vi "Main.vi"() -> ()   [LabVIEW 2019, in "TemplateModule.lvlib"]
doc: "This VI is a template for all GUI VIs in TMOS. Be careful with colours, they may require updating."
uses:
  TemplateModule.lvlib
  Gui/Gui.TopBar.ctl
  Tools/controls/buttons/OK.ctl
  Tools/controls/buttons/Cancel.ctl
  Tools/controls/buttons/Reload.ctl
  Tools/controls/buttons/Save.ctl
  Action.ctl
  Gui/Gui.TopBar.Visibility.ctl
  Tools/CitTemplate/citTemplate.errData.ctl
  Tools/Tools.lvlib
panel:
  in  "Module top bar":T1
  # "version: 1.0"
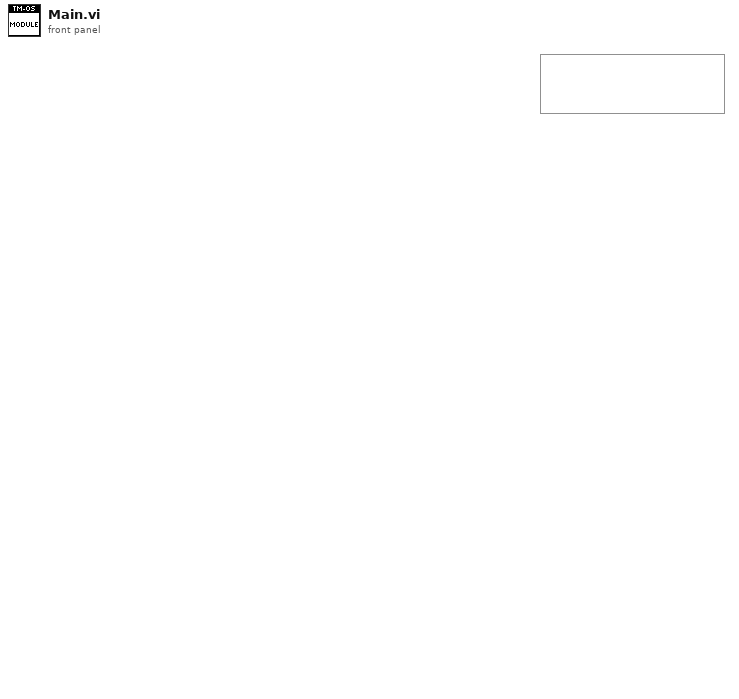
[diagram p1: front panel]
types:
  T1 = typedef "TemplateModule.lvlib/Gui.TopBar.ctl" = cluster{"OK":T2, "Cancel":T3, "Reload":T4, "Save":T5, "Module name":string}
  T2 = typedef "Tools.lvlib/OK.ctl" = bool
  T3 = typedef "Tools.lvlib/Cancel.ctl" = bool
  T4 = typedef "Tools.lvlib/Reload.ctl" = bool
  T5 = typedef "Tools.lvlib/Save.ctl" = bool
  T6 = typedef "TemplateModule.lvlib/Action.ctl" = enum32{"idle", "constructor", "destructor", "--- Module.Gui ---", "Translate.Gui", "update"}
  T7 = typedef "Tools.lvlib/citTemplate.errData.ctl" = cluster{"action":string, "error":errorcluster}
  T8 = typedef "Tools.lvlib/citTemplate.notifierHandle.ctl" = refnum<notifier>
  T9 = typedef "TemplateModule.lvlib/Gui.TopBar.Visibility.ctl" = cluster{"OK":bool, "Cancel":bool, "Reload":bool, "Save":bool, "Module name":bool}
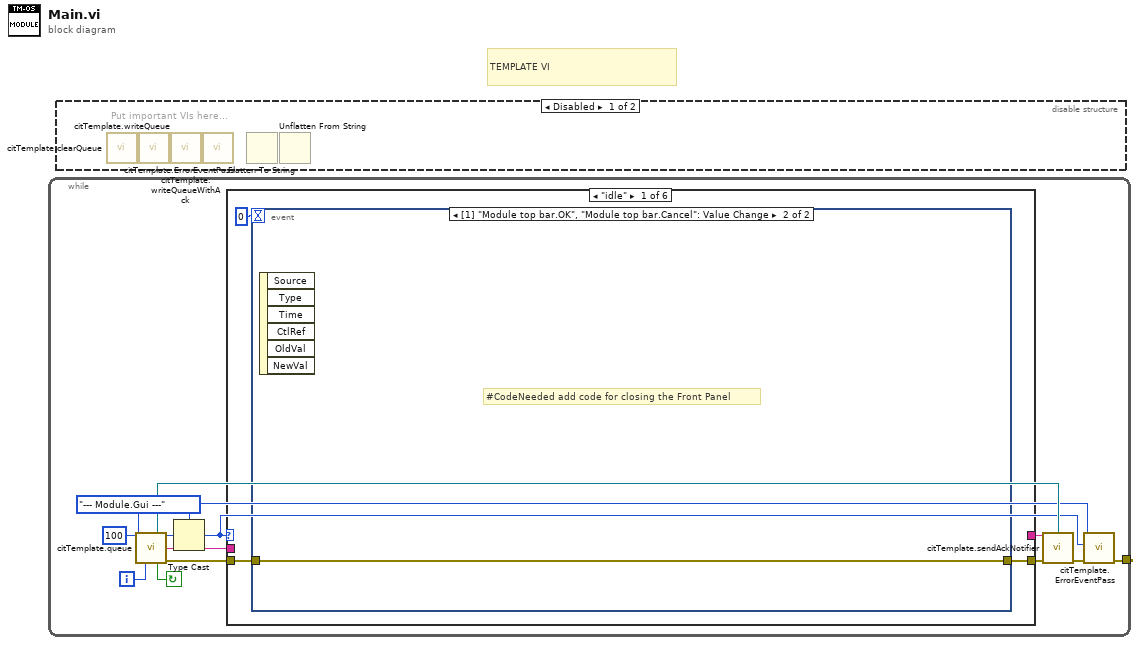
[diagram p0: block diagram]
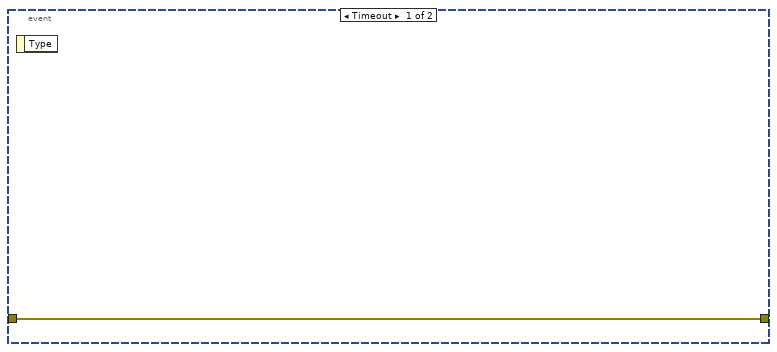
[diagram p3: hidden frame]
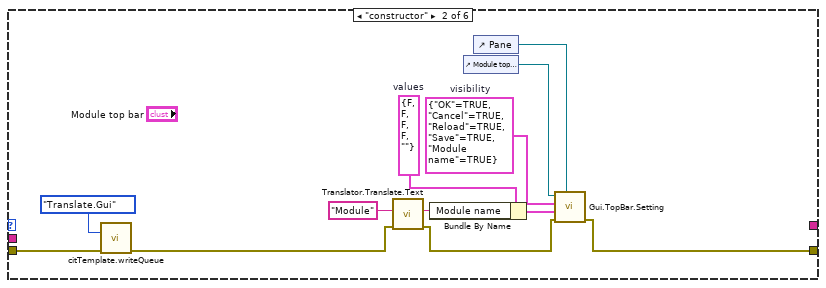
[diagram p4: hidden frame]
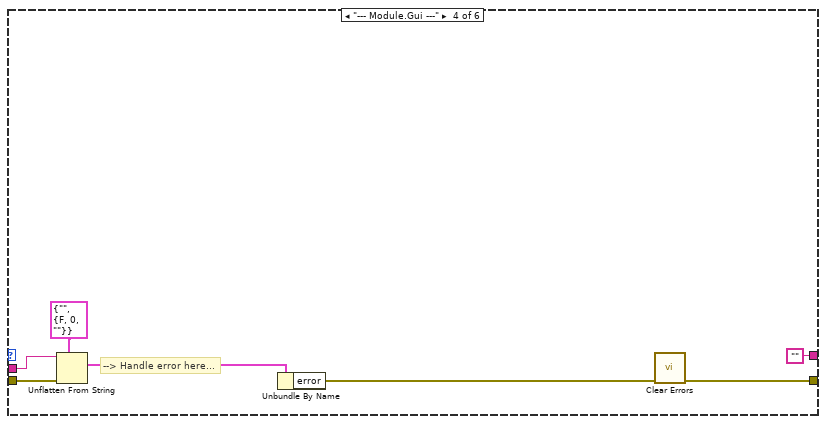
[diagram p6: hidden frame]
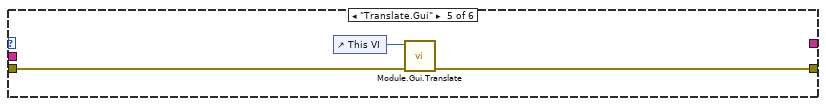
[diagram p7: hidden frame]
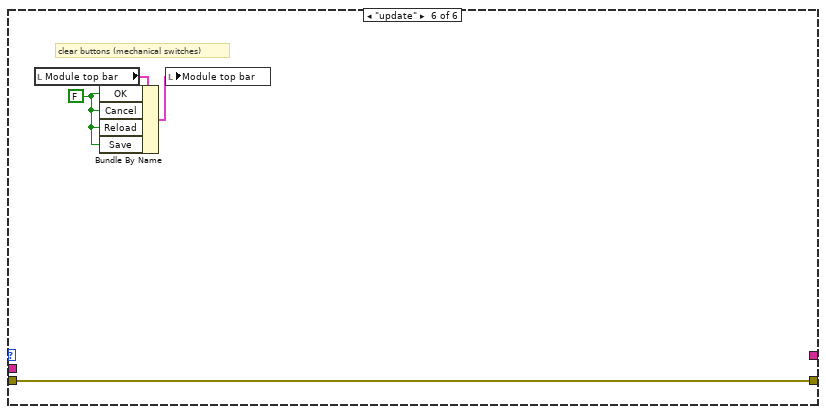
[diagram p8: hidden frame]
diagram:
  # "TEMPLATE VI"
  n1 = while {
    tunnel: [w2] -> _
    i -> [w8]
    stop <- w9 continue-if-true
    w1 = Action."--- Module.Gui ---" ("Action")
    n2 = call "citTemplate.queue.vi"("ms timeout (250 ms)"=100, "event enum"=w1, "iteration (-1)"=w8) -> ("notifierHandle out"=w6:T8, "event out"=w12:u32, "(flatten) data out"=w11:string, "continue"=w9:bool, "error out"=w10:errorcluster)  [unwired: 2 in, 6 out]
    n3 = Type Cast(type=w1, x=w12) -> (*(type *) &x=w3:T6)
    n4 = case shown="\"idle\"" w3 {
      tunnel: w11 -> [_ _ _ w37 _ _]
      tunnel: w10 -> [w14 w29 w30 w36 w39 w44]
      tunnel: [w13 w22 w30 w34 w38 w44] -> w4
      tunnel: [_ _ _ "" _ _] -> w5
      frame "idle" {
        n5 = event shown="[1] \"Module top bar.OK\", \"Module top bar.Cancel\": Value Change" {
          selector: _ -> [_ _]
          dyn-events: _ -> [_ _]
          timeout: 0 -> [_ _]
          tunnel: [w16 w17] -> w13
          tunnel: w14 -> [w16 w17]
          event Timeout {
            n6 = event-data() -> ()  [unwired: 1 in, 1 out]
          }
          event Value Change {
            # "#CodeNeeded add code for closing the Front Panel"
            n7 = event-data() -> ()  [unwired: 1 in, 6 out]
          }
        }
      }
      frame "constructor" {
        w26 = T1 {"OK"=FALSE, "Cancel"=FALSE, "Reload"=FALSE, "Save"=FALSE, "Module name"=""}  # values
        w27 = T9 {"OK"=TRUE, "Cancel"=TRUE, "Reload"=TRUE, "Save"=TRUE, "Module name"=TRUE}  # visibility
        n8 = call "citTemplate.writeQueue.vi"("event in (if not connected:all statemachine with data event)"=Action."Translate.Gui" ("Action"), "error in (no error)"=w29) -> ("error out"=w23:errorcluster)  [unwired: 13 in]
        n9 = call "Translator.Translate.Text.vi"("error in"=w23, "text"="Module" ("Module name")) -> ("error out"=w21:errorcluster, "translated text"=w24:string)  [unwired: 8 in]
        n10 = Bundle By Name(cluster=w26, "Module name"=w24) -> (w25:T1)
        n11 = control-ref of="Module top bar"() -> (w18:refnum<vi>)
        n12 = control-ref of="Pane"() -> (w19:refnum<vi>)
        n13 = call "Gui.TopBar.Setting.vi"("pane ref in"=w19, "error in"=w21, "values"=w25, "visibility"=w27, "top bar ref in"=w18) -> ("error out"=w22:errorcluster)  [unwired: 5 in, 1 out]
      }
      frame "destructor" {
      }
      frame "--- Module.Gui ---" {
        # "--> Handle error here..."
        n14 = Unflatten From String(type=T7 {"action"="", "error"={"status"=FALSE, "code"=0, "source"=""}} ("ErrData"), binary string=w37, error in (no error)=w36) -> (value=w35:T7)  [unwired: 4 out]
        n15 = Unbundle By Name(w35) -> ("error"=w31:errorcluster)
        n16 = call <vilib>:"Clear Errors.vi"("error in (no error)"=w31) -> ("error out"=w34:errorcluster)  [unwired: 5 in, 1 out]
      }
      frame "Translate.Gui" {
        n17 = control-ref of="This VI"() -> (w40:refnum<vi>)
        n18 = call "Module.Gui.Translate.vi"("error in"=w39, "VI ref in"=w40) -> ("error out"=w38:errorcluster)  [unwired: 7 in, 2 out]
      }
      frame "update" {
        w42 = FALSE ("OK")
        # "clear buttons (mechanical switches)"
        n19 = local read "Module top bar"() -> (w43:T1)
        n20 = Bundle By Name(cluster=w43, "OK"=w42, "Cancel"=w42, "Reload"=w42, "Save"=w42) -> (w41:T1)
        n21 = local write "Module top bar"(w41) -> ()
      }
    }
    n22 = call "citTemplate.sendAckNotifier.vi"("notification data"=w5, "notifierHandle in"=w6, "error in"=w4) -> ()  [unwired: 13 in]
    n23 = call "citTemplate.ErrorEventPass.vi"("error in (no error)"=w4, "action of error"=w3, "event in"=w1) -> ("error out"=w2:errorcluster)  [unwired: 8 in]
  }
  n24 = disable-structure shown="Disabled" {
    frame Disabled {
      # "Put important VIs here..."
      n25 = call "citTemplate.clearQueue.vi"() -> ()  [unwired: 14 in, 2 out]
      n26 = call "citTemplate.writeQueue.vi"() -> ()  [unwired: 15 in, 1 out]
      n27 = call "citTemplate.writeQueueWithAck.vi"() -> ()  [unwired: 13 in, 3 out]
      n28 = call "citTemplate.ErrorEventPass.vi"() -> ()  [unwired: 11 in, 1 out]
      n29 = Flatten To String() -> ()  [unwired: 4 in, 3 out]
      n30 = Unflatten From String() -> ()  [unwired: 5 in, 3 out]
    }
    frame Enabled {
    }
  }
